vi "Apply PID Parameters.vi"(10 "Parameters in":T1 {"Config"."Industrial Settings"."Write Refs"."Data Reference" format="%.0x"; "Config"."Industrial Settings"."Read Refs"."Data Reference" format="%.0x"; "Config"."PID Settings"."Read Refs"."Data Reference" format="%.0x"; "Config"."PID Settings"."Write Refs"."Data Reference" format="%.0x"}, 11 "UpdateParameters":T9) -> (2 "Parameters out":T1 {"Config"."Industrial Settings"."Write Refs"."Data Reference" format="%.0x"; "Config"."Industrial Settings"."Read Refs"."Data Reference" format="%.0x"; "Config"."PID Settings"."Read Refs"."Data Reference" format="%.0x"; "Config"."PID Settings"."Write Refs"."Data Reference" format="%.0x"})   [LabVIEW 2019, in "Control Addon Engine.lvlib"]
uses:
  Control Addon Engine.lvlib
  Types/RT Configuration.ctl
  Shared/Types/Gain Schedule.ctl
  Shared/Types/Compiled Settings.ctl
  Shared/Types/Compiled PID Settings.ctl
  <vilib>/NI VeriStand/Custom Device API/Block Data Reference.ctl
  <vilib>/NI VeriStand/Custom Device API/Data Reference.ctl
  Shared/Types/Compiled Industrial Settings.ctl
  Shared/Types/Compiled Industrial Parameters.ctl
  Shared/Types/Update Parameters Message.ctl
  Shared/Control Addon Shared.lvlib
  <vilib>/NI VeriStand/Custom Device API/Custom Device API.lvlib
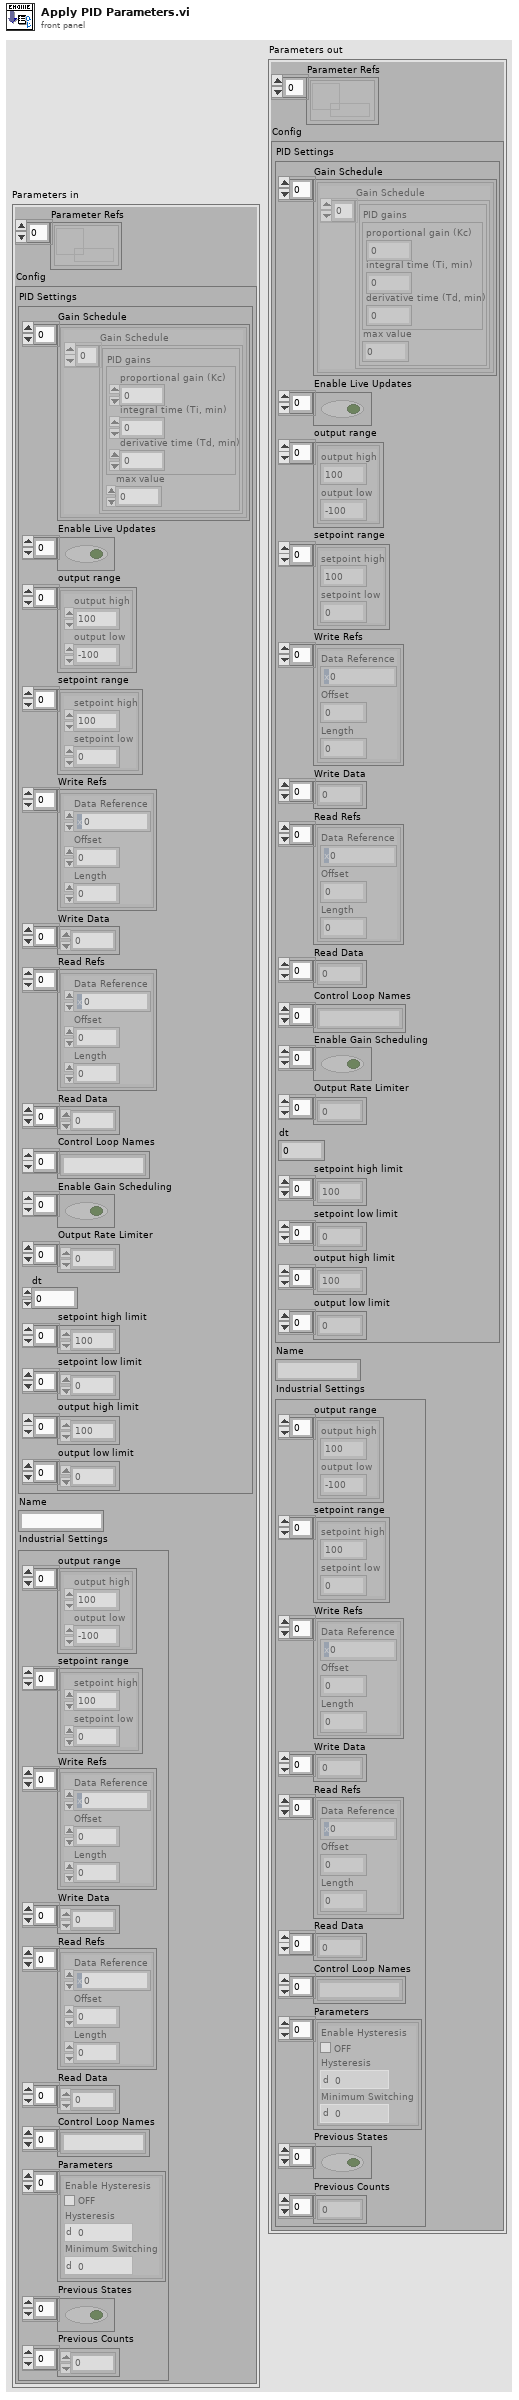
[diagram p1: front panel]
types:
  T1 = typedef "Control Addon Engine.lvlib/RT Configuration.ctl" = cluster{"Parameter Refs":refnum<data-value>[], "Config":T2}
  T2 = typedef "Control Addon Shared.lvlib/Compiled Settings.ctl" = cluster{"PID Settings":T3, "Name":string, "Industrial Settings":T7}
  T3 = typedef "Control Addon Shared.lvlib/Compiled PID Settings.ctl" = cluster{"Gain Schedule":T4[], "Enable Live Updates":bool[], "output range":cluster{"output high":dbl, "output low":dbl}[], "setpoint range":cluster{"setpoint high":dbl, "setpoint low":dbl}[], "Write Refs":T5[], "Write Data":dbl[], "Read Refs":T5[], "Read Data":dbl[], "Control Loop Names":string[], "Enable Gain Scheduling":bool[], "Output Rate Limiter":dbl[], "dt":dbl, "setpoint high limit":dbl[], "setpoint low limit":dbl[], "output high limit":dbl[], "output low limit":dbl[]}
  T4 = typedef "Control Addon Shared.lvlib/Gain Schedule.ctl" = cluster{"Gain Schedule":cluster{"PID gains":cluster{"proportional gain (Kc)":dbl, "integral time (Ti, min)":dbl, "derivative time (Td, min)":dbl}, "max value":dbl}[]}
  T5 = typedef "Custom Device API.lvlib/Block Data Reference.ctl" = cluster{"Data Reference":T6, "Offset":u64, "Length":u64}
  T6 = typedef "Custom Device API.lvlib/Data Reference.ctl" = i32
  T7 = typedef "Control Addon Shared.lvlib/Compiled Industrial Settings.ctl" = cluster{"output range":cluster{"output high":dbl, "output low":dbl}[], "setpoint range":cluster{"setpoint high":dbl, "setpoint low":dbl}[], "Write Refs":T5[], "Write Data":dbl[], "Read Refs":T5[], "Read Data":dbl[], "Control Loop Names":string[], "Parameters":T8[], "Previous States":bool[], "Previous Counts":u64[]}
  T8 = typedef "Control Addon Shared.lvlib/Compiled Industrial Parameters.ctl" = cluster{"Enable Hysteresis":bool, "Hysteresis":dbl, "Minimum Switching":u64}
  T9 = typedef "Control Addon Shared.lvlib/Update Parameters Message.ctl" = cluster{"Control Loop":string, "Gain Schedule":cluster{"PID gains":cluster{"proportional gain (Kc)":dbl, "integral time (Ti, min)":dbl, "derivative time (Td, min)":dbl}, "max value":dbl}[]}
  T10 = cluster{"PID gains":cluster{"proportional gain (Kc)":dbl, "integral time (Ti, min)":dbl, "derivative time (Td, min)":dbl}, "max value":dbl}[]
  T11 = typedef "Simple PID Addon Shared.lvlib/Gain Schedule.ctl" = cluster{"Gain Schedule":cluster{"PID gains":cluster{"proportional gain (Kc)":dbl, "integral time (Ti, min)":dbl, "derivative time (Td, min)":dbl}, "max value":dbl}[]}
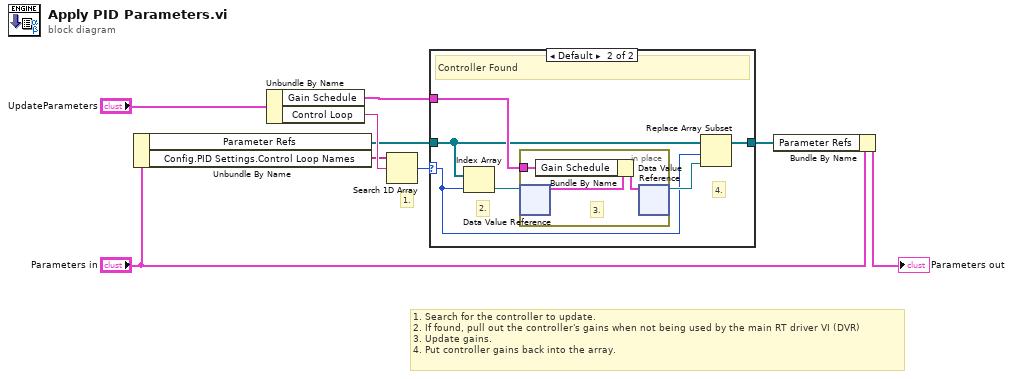
[diagram p0: block diagram]
diagram:
  # "1. Search for the controller to update.\n2. If found, pull out the controller's gains when not being used by the main RT driver VI (DVR)\n3. Update gains.\n4. Put controller gains back into the array."
  # "1."
  n1 = Unbundle By Name("Parameters in") -> ("Parameter Refs"=w3:refnum<data-value>[], "Config.PID Settings.Control Loop Names"=w2:string[])
  n2 = Unbundle By Name("UpdateParameters") -> ("Gain Schedule"=w8:T10, "Control Loop"=w7:string)
  n3 = Search 1D Array(1D array=w2, element=w7) -> (index of element=w1:i32)  [unwired: 1 in]
  n4 = case shown="Default" w1 {
    selector: w1 -> [_ w11]
    tunnel: w8 -> [_ w16]
    tunnel: [w10 w15] -> w5
    tunnel: w3 -> [w10 w14]
    frame -1 {
      # "Controller not found"
    }
    frame Default {
      # "4."
      # "2."
      # "Controller Found"
      n5 = Index Array(array=w14, index=w11) -> (element=w12:refnum<data-value>)
      n6 = in-place {
        in-place-border: w16 -> [w17]
        # "3."
        n7 = in-place-dvr #1(w12) -> (w19:T11)  [unwired: 1 out]
        n8 = Bundle By Name(cluster=w19, "Gain Schedule"=w17) -> (w18:T11)
        n9 = in-place-dvr #1(w18) -> (w13:refnum<data-value>)  [unwired: 1 out]
      }
      n10 = Replace Array Subset(array=w14, new element=w13, index=w11) -> (w15:refnum<data-value>[])
    }
  }
  n11 = Bundle By Name(cluster="Parameters in", "Parameter Refs"=w5) -> (→"Parameters out":T1)
